vi "GrabberArms Controller.vi"(8 "error in (no error)":errorcluster, 11 "Extend GrabberArms":bool) -> (0 "error out":errorcluster)   [LabVIEW 2013]
uses:
  Systems/GrabberArms/GrabberArms.lvclass
  Robot Global Data.vi
  Commands/GA-Extend-Command/GA-Extend-Cmd.lvclass
  Commands/GA-Retract-Command/GA-Retract-Cmd.lvclass
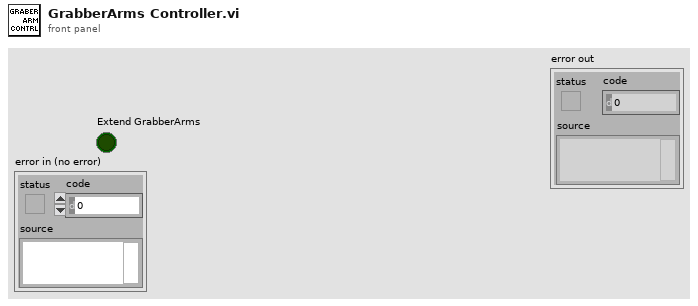
[diagram p1: front panel]
types:
  T1 = typedef "Semaphore RefNum" = refnum<k1>
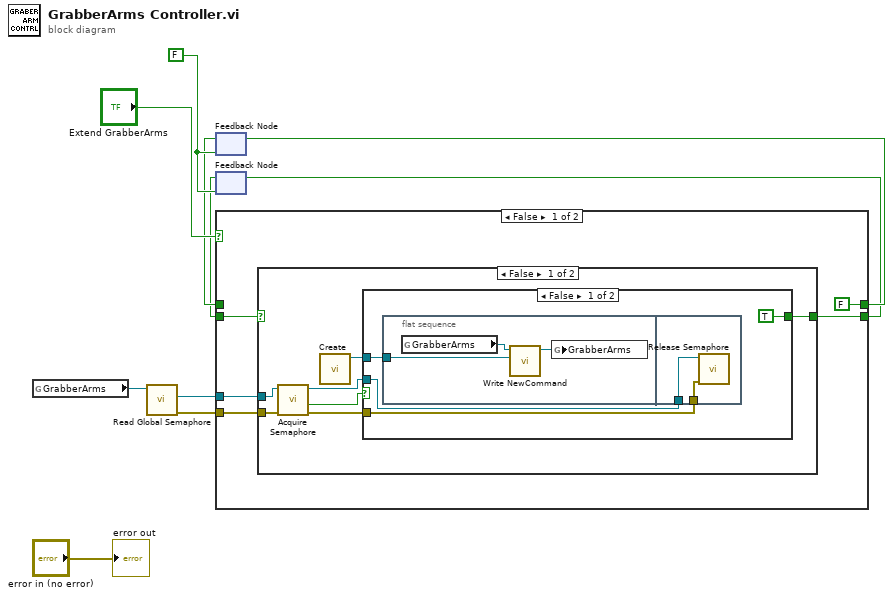
[diagram p0: block diagram]
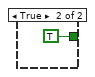
[diagram p2: hidden frame]
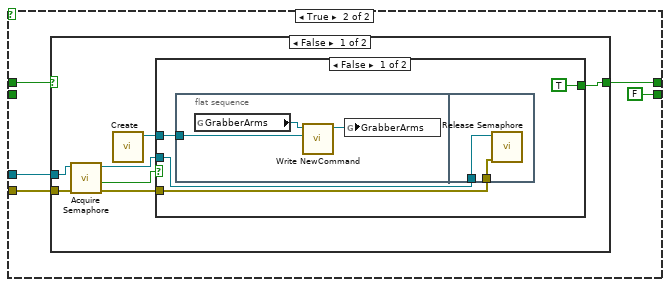
[diagram p4: hidden frame]
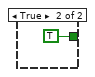
[diagram p5: hidden frame]
diagram:
  w9 = FALSE
  n1 = global read "Robot Global Data.vi" "GrabberArms"() -> (w6:refnum<class "GrabberArms.lvclass">)
  n2 = call-dynamic "Read Global Semaphore.vi"("System in"=w6) -> ("error out"=w4:errorcluster, "semaphore"=w5:T1)  [unwired: 8 in, 1 out]
  n3 = feedback #1(w9) -> (w8:bool)
  n4 = feedback #2(w9) -> (w2:bool)
  n5 = case shown="False" "Extend GrabberArms" {
    tunnel: w8 -> [_ w38]
    tunnel: [FALSE w37] -> w7
    tunnel: w5 -> [w15 w36]
    tunnel: w4 -> [w14 w35]
    tunnel: [w13 FALSE] -> w3
    tunnel: w2 -> [w11 _]
    frame False {
      n6 = case shown="False" w11 {
        selector: w11 -> [_ w33]
        tunnel: [w16 w33] -> w13
        tunnel: w15 -> [w22 _]
        tunnel: w14 -> [w21 _]
        frame False {
          n7 = call <vilib>:"Acquire Semaphore.vi"("error in (no error)"=w21, "semaphore"=w22) -> ("error out"=w20:errorcluster, "timed out"=w17:bool, "semaphore out"=w19:T1)  [unwired: 3 in]
          n8 = call "Create.vi"() -> ("GA-Retract-Cmd out"=w18:refnum<class "GA-Retract-Cmd.lvclass">)  [unwired: 10 in, 1 out]
          n9 = case shown="False" w17 {
            tunnel: w20 -> [w26 _]
            tunnel: w19 -> [w25 _]
            tunnel: w18 -> [w24 _]
            tunnel: [TRUE TRUE] -> w16
            frame False {
              n10 = flat-sequence {
                tunnel: w24 -> [w27]
                tunnel: w26 -> [w31]
                tunnel: w25 -> [w30]
                frame #0 {
                  n11 = global read "Robot Global Data.vi" "GrabberArms"() -> (w29:refnum<class "GrabberArms.lvclass">)
                  n12 = call-dynamic "Write NewCommand.vi"("Command.lvclass"=w27, "System in"=w29) -> ("System out"=w28:refnum<class "GrabberArms.lvclass">)  [unwired: 8 in, 1 out]
                  n13 = global write "Robot Global Data.vi" "GrabberArms"(w28) -> ()
                }
                frame #1 {
                  n14 = call <vilib>:"Release Semaphore.vi"("error in (no error)"=w31, "semaphore"=w30) -> ()  [unwired: 4 in, 2 out]
                }
              }
            }
            frame True {
            }
          }
        }
        frame True {
        }
      }
    }
    frame True {
      n15 = case shown="False" w38 {
        selector: w38 -> [_ w56]
        tunnel: [w39 w56] -> w37
        tunnel: w36 -> [w45 _]
        tunnel: w35 -> [w44 _]
        frame False {
          n16 = call <vilib>:"Acquire Semaphore.vi"("error in (no error)"=w44, "semaphore"=w45) -> ("error out"=w43:errorcluster, "timed out"=w40:bool, "semaphore out"=w42:T1)  [unwired: 3 in]
          n17 = call "Create.vi"() -> ("GA-Extend-Cmd out"=w41:refnum<class "GA-Extend-Cmd.lvclass">)  [unwired: 10 in, 1 out]
          n18 = case shown="False" w40 {
            tunnel: w43 -> [w49 _]
            tunnel: w42 -> [w48 _]
            tunnel: w41 -> [w47 _]
            tunnel: [TRUE TRUE] -> w39
            frame False {
              n19 = flat-sequence {
                tunnel: w47 -> [w50]
                tunnel: w49 -> [w54]
                tunnel: w48 -> [w53]
                frame #0 {
                  n20 = global read "Robot Global Data.vi" "GrabberArms"() -> (w52:refnum<class "GrabberArms.lvclass">)
                  n21 = call-dynamic "Write NewCommand.vi"("Command.lvclass"=w50, "System in"=w52) -> ("System out"=w51:refnum<class "GrabberArms.lvclass">)  [unwired: 8 in, 1 out]
                  n22 = global write "Robot Global Data.vi" "GrabberArms"(w51) -> ()
                }
                frame #1 {
                  n23 = call <vilib>:"Release Semaphore.vi"("error in (no error)"=w54, "semaphore"=w53) -> ()  [unwired: 4 in, 2 out]
                }
              }
            }
            frame True {
            }
          }
        }
        frame True {
        }
      }
    }
  }
  n24 = feedback-in #1(w7) -> ()
  n25 = feedback-in #2(w3) -> ()
  "error out" <- "error in (no error)"
